vi "automated_sleep_detection_mode.vi"(5 "Input \nparameters":T3={"Frame rate (ms)"=2000, "Worm strain"="N2", "# Images"=0, "State"=enum."Image acquisition", "Time elapsed"=0.0, "Max_num_runs"=100000, "#TTL"=0, "Time of start TTL"=100000, "ImSub Value"=0, "Time of last TTL"=0, "Number of Columns"=2, "Number of Rows"=2, "# AdjacentTTL"=0, "Sleep deprivation status"="", "Sleep Detection"=FALSE, "# Sleep detections"=0, "Time of first sleep detection"=0, "Time max # adjacent TTL"=0, "Image t-1"=[], "Image t"=[]} {"Number of Rows" items=["1"=1, "2"=2, "3"=3, "4"=4]; "Number of Columns" items=["1"=1, "2"=2, "3"=3, "4"=4]}, 6 "Deprivation\nparameters":T1={"Frame Row"=0, "Kstd"=40.0, "# Images for\nsleep detection"=10, "Kmean"=1.5, "Start time of sleep detection"=1000, 0, "Max deprivation length"=3600, "Max # TTL"=10000, "Delay detection start by x images after first detection"=0, "Minimum Interval between TTL pulses"=0, "Delay sleep detection\nby x detections"=9, "# Total immobility detections"=0, "Pause max # adjacent\nTTL"=0, "TTL x start\ntime deprivation\n"=0.0, "Max #\nadjacent TTL"=10000, " Ca2+\nmode"=0} {"?" items=["1", "2", "3", "4"]; "Frame Row" items=["1", "2", "3", "4"]}) -> (1 "Output \nparameters":T4={"Frame rate (ms)"=2000, "Worm strain"="N2", "Time t"=0, "State"=enum."Image acquisition", "Time elapsed"=0.0, "Max_num_runs"=100000, "#TTL"=0, "Time of start TTL"=100000, "ImSub Value"=0, "Time of last TTL"=0, "Number of Columns"=2, "Number of Rows"=2, "# AdjacentTTL"=0, "Sleep deprivation status"="", "Sleep Detection"=FALSE, "# Sleep detections"=0, "Time of first sleep detection"=0, "Time max # adjacent TTL"=0, "Image t-1"=[], "Image t"=[]} {"Number of Rows" items=["1"=1, "2"=2, "3"=3, "4"=4]; "Number of Columns" items=["1"=1, "2"=2, "3"=3, "4"=4]})   [LabVIEW 2011]
uses:
  state.ctl
  Action-Init-Update-Get.ctl
panel:
  # "Sleep deprivation settings"
  # "Select deprivation animal"
  # "Deprive image in row"
  # "Deprive image in column"
  # "Sleep detection parameters"
  # "Sleep deprivation parameters"
  # "Delay deprivation start:"
  # "Pause deprivation (images):"
  # "Stop deprivation after:"
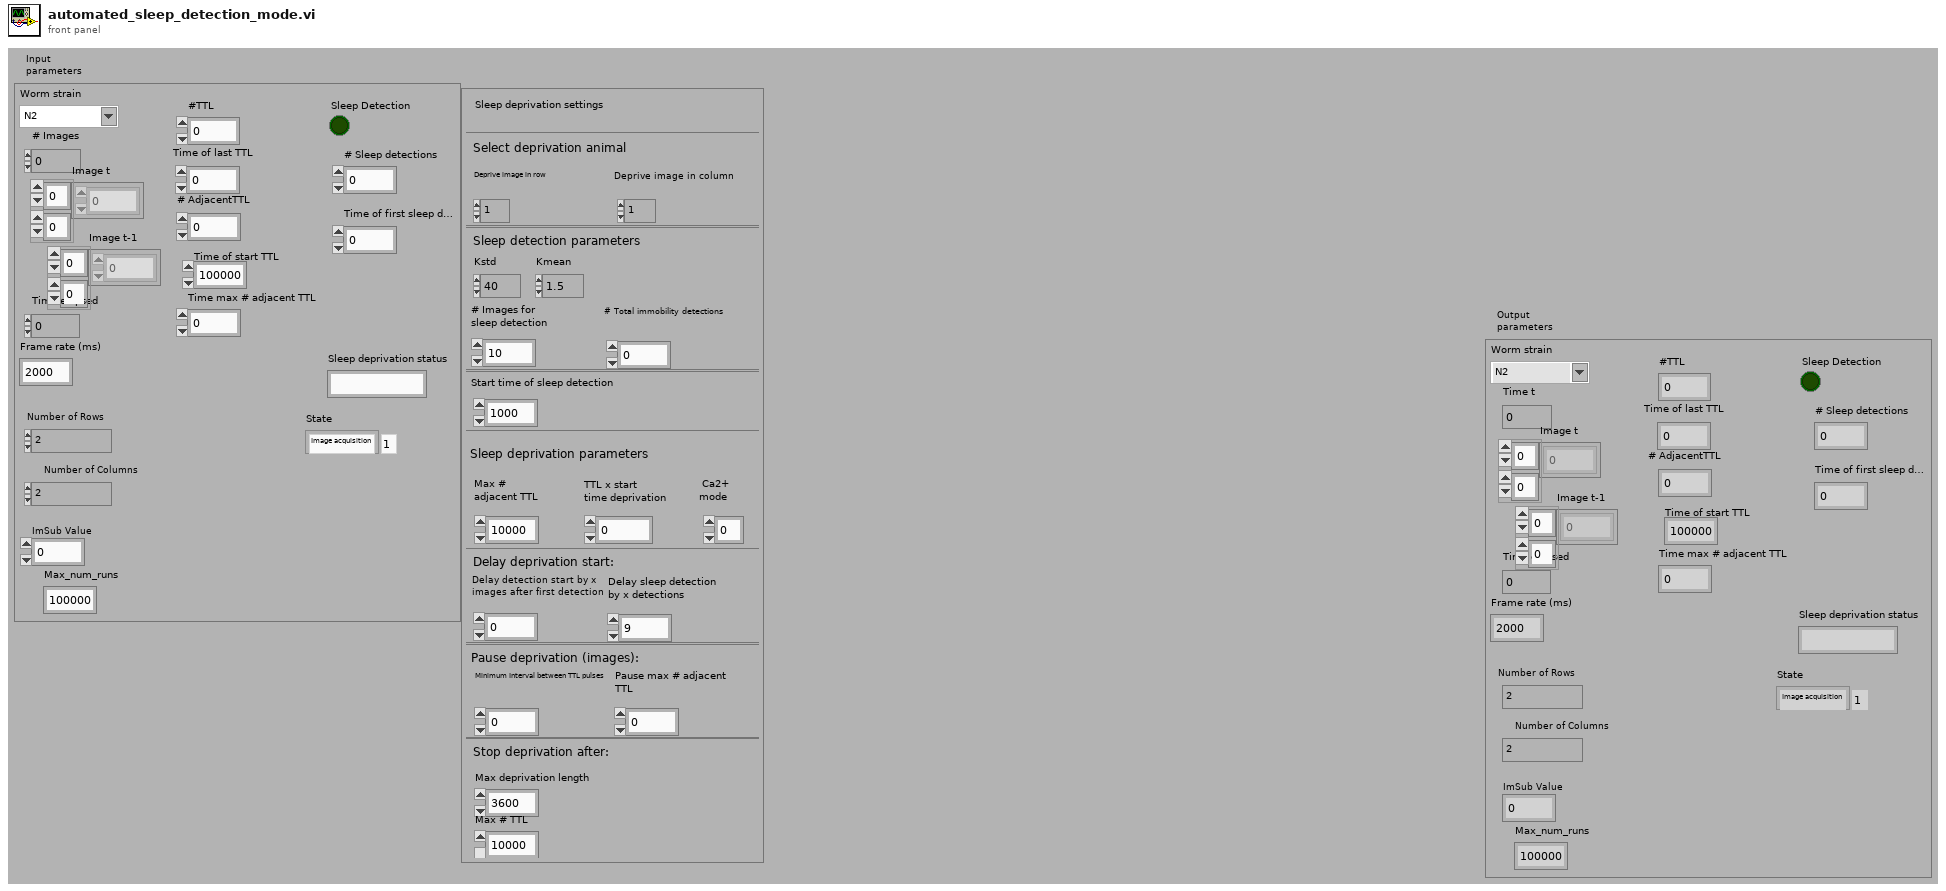
[diagram p1: front panel]
types:
  T1 = cluster{"Frame Row":u32, "Kstd":dbl, "# Images for\nsleep detection":i32, "Kmean":dbl, "Start time of sleep detection":i32, u32, "Max deprivation length":i32, "Max # TTL":i32, "Delay detection start by x images after first detection":i32, "Minimum Interval between TTL pulses":i32, "Delay sleep detection\nby x detections":i32, "# Total immobility detections":i32, "Pause max # adjacent\nTTL":i32, "TTL x start\ntime deprivation\n":dbl, "Max #\nadjacent TTL":i32, " Ca2+\nmode":i32}
  T2 = typedef "state.ctl" = enum16{"Initialize measurement", "Image acquisition", "Image processing", "Sleep detection", "Control TTL protocol ", "Sleep deprivation", "Update image & exit condition", "Wait "}
  T3 = cluster{"Frame rate (ms)":u32, "Worm strain":string, "# Images":i32, "State":T2, "Time elapsed":dbl, "Max_num_runs":i32, "#TTL":i32, "Time of start TTL":i32, "ImSub Value":i32, "Time of last TTL":i32, "Number of Columns":u32, "Number of Rows":u32, "# AdjacentTTL":i32, "Sleep deprivation status":string, "Sleep Detection":bool, "# Sleep detections":i32, "Time of first sleep detection":i32, "Time max # adjacent TTL":i32, "Image t-1":i32[][], "Image t":i32[][]}
  T4 = cluster{"Frame rate (ms)":u32, "Worm strain":string, "Time t":i32, "State":T2, "Time elapsed":dbl, "Max_num_runs":i32, "#TTL":i32, "Time of start TTL":i32, "ImSub Value":i32, "Time of last TTL":i32, "Number of Columns":u32, "Number of Rows":u32, "# AdjacentTTL":i32, "Sleep deprivation status":string, "Sleep Detection":bool, "# Sleep detections":i32, "Time of first sleep detection":i32, "Time max # adjacent TTL":i32, "Image t-1":i32[][], "Image t":i32[][]}
  T5 = typedef "Action-Init-Update-Get.ctl" = enum16{"Initialize", "Update", "Get"}
  T6 = cluster{"Global image subtraction array":dbl[], "Local image subtraction array":dbl[]}
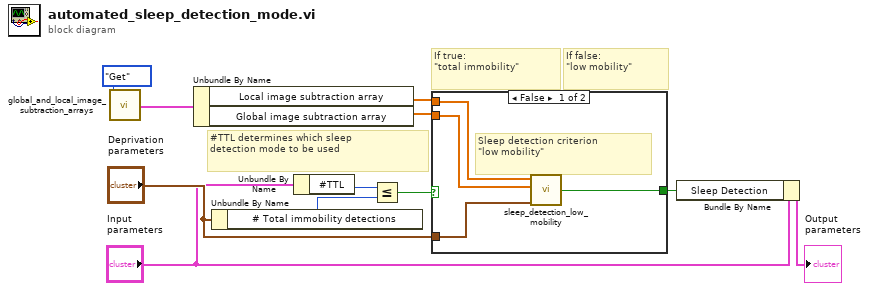
[diagram p0: block diagram]
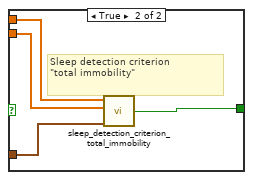
[diagram p2: hidden frame]
diagram:
  # "#TTL determines which sleep \ndetection mode to be used"
  # "If false:\n\"low mobility\""
  # "If true:\n\"total immobility\""
  n1 = call "global_and_local_image_subtraction_arrays.vi"("State"=Action-Init-Update-Get."Get" ("Action")) -> ("Image subtraction\narrays"=w4:T6)  [unwired: 10 in]
  n2 = Unbundle By Name(w4) -> ("Local image subtraction array"=w3:dbl[], "Global image subtraction array"=w2:dbl[])
  n3 = Unbundle By Name("Deprivation\nparameters") -> ("# Total immobility detections"=w9:i32)
  n4 = Unbundle By Name("Input \nparameters") -> ("#TTL"=w10:i32)
  n5 = Less Or Equal?(x=w10, y=w9) -> (x <= y?=w11:bool)
  n6 = case shown="False" w11 {
    tunnel: w3 -> [w15 w19]
    tunnel: w2 -> [w14 w18]
    tunnel: [w12 w16] -> w8
    tunnel: "Deprivation\nparameters" -> [w13 w17]
    frame False {
      # "Sleep detection criterion\n\"low mobility\""
      n7 = call "sleep_detection_low_mobility.vi"("Deprivation\nparameters"=w13, "Global image \nsubtraction array"=w14, "Local image \nsubtraction array"=w15) -> ("Sleep detection"=w12:bool)  [unwired: 8 in]
    }
    frame True {
      # "Sleep detection criterion\n\"total immobility\""
      n8 = call "sleep_detection_criterion_total_immobility.vi"("Deprivation\nparameters"=w17, "Global image \nsubtraction array"=w18, "Local image \nsubtraction array"=w19) -> ("Sleep detection"=w16:bool)  [unwired: 3 in]
    }
  }
  n9 = Bundle By Name(cluster="Input \nparameters", "Sleep Detection"=w8) -> (→"Output \nparameters":T3)
